vi "Lab Panel V5.12.vi"() -> ()   [LabVIEW 2013] (continued)
              n217 = local read "TEMP LA02"() -> (w247:T9)
              n218 = Bundle By Name(cluster=w247, "TL-1"=w239, "TN-1"=w238, "TL-2"=w237, "TN-2"=w236, "TL -1COUNT"=w244, "TN-1 COUNT"=w244, "TL-2 COUNT"=w244, "TN-2 COUNT"=w244) -> (w245:T9)
              n219 = Bundle(cluster=w242, "Tmp Live"=w237, "Tmp Neut"=w236) -> (w240:T2)  [unwired: 3 in]
              n220 = Bundle(cluster=w243, "Tmp Live"=w239, "Tmp Neut"=w238) -> (w241:T2)  [unwired: 3 in]
              n221 = local write "TEMP LA02"(w245) -> ()
              n222 = local write "SIG LAB02-1"(w241) -> ()
              n223 = local write "SIG LAB02-2"(w240) -> ()
            }
            frame #4 {
              w256 = 0
              n224 = local read "LAB03 TEMP"() -> (w258:T12)
              n225 = Unbundle By Name(w258) -> ("T1 Live"=w251:dbl, "T1 Neut"=w250:dbl, "T2 Live"=w249:dbl, "T2 Neut"=w248:dbl)  [unwired: 2 out]
              n226 = local read "SIG LAB03-1"() -> (w255:T2)
              n227 = local read "SIG LAB03-2"() -> (w254:T2)
              n228 = local read "TEMP LA03"() -> (w259:T9)
              n229 = Bundle By Name(cluster=w259, "TL-1"=w251, "TN-1"=w250, "TL-2"=w249, "TN-2"=w248, "TL -1COUNT"=w256, "TN-1 COUNT"=w256, "TL-2 COUNT"=w256, "TN-2 COUNT"=w256) -> (w257:T9)
              n230 = Bundle(cluster=w254, "Tmp Live"=w249, "Tmp Neut"=w248) -> (w252:T2)  [unwired: 3 in]
              n231 = Bundle(cluster=w255, "Tmp Live"=w251, "Tmp Neut"=w250) -> (w253:T2)  [unwired: 3 in]
              n232 = local write "TEMP LA03"(w257) -> ()
              n233 = local write "SIG LAB03-2"(w252) -> ()
              n234 = local write "SIG LAB03-1"(w253) -> ()
            }
            frame #5 {
              w268 = 0
              n235 = local read "LAB04 TEMP"() -> (w270:T12)
              n236 = Unbundle By Name(w270) -> ("T1 Live"=w263:dbl, "T1 Neut"=w262:dbl, "T2 Live"=w261:dbl, "T2 Neut"=w260:dbl)  [unwired: 2 out]
              n237 = local read "SIG LAB04-2"() -> (w266:T2)
              n238 = local read "SIG LAB04-1"() -> (w267:T2)
              n239 = local read "TEMP LA04"() -> (w271:T9)
              n240 = Bundle By Name(cluster=w271, "TL-1"=w263, "TN-1"=w262, "TL-2"=w261, "TN-2"=w260, "TL -1COUNT"=w268, "TN-1 COUNT"=w268, "TL-2 COUNT"=w268, "TN-2 COUNT"=w268) -> (w269:T9)
              n241 = Bundle(cluster=w266, "Tmp Live"=w261, "Tmp Neut"=w260) -> (w264:T2)  [unwired: 3 in]
              n242 = Bundle(cluster=w267, "Tmp Live"=w263, "Tmp Neut"=w262) -> (w265:T2)  [unwired: 3 in]
              n243 = local write "SIG LAB04-2"(w264) -> ()
              n244 = local write "TEMP LA04"(w269) -> ()
              n245 = local write "SIG LAB04-1"(w265) -> ()
            }
            frame #6 {
              w280 = 0
              n246 = local read "LAB05 TEMP"() -> (w282:T12)
              n247 = Unbundle By Name(w282) -> ("T1 Live"=w275:dbl, "T1 Neut"=w274:dbl, "T2 Live"=w273:dbl, "T2 Neut"=w272:dbl)  [unwired: 2 out]
              n248 = local read "SIG LAB05-2"() -> (w278:T2)
              n249 = local read "SIG LAB05-1"() -> (w279:T2)
              n250 = local read "TEMP LA05"() -> (w283:T9)
              n251 = Bundle By Name(cluster=w283, "TL-1"=w275, "TN-1"=w274, "TL-2"=w273, "TN-2"=w272, "TL -1COUNT"=w280, "TN-1 COUNT"=w280, "TL-2 COUNT"=w280, "TN-2 COUNT"=w280) -> (w281:T9)
              n252 = Bundle(cluster=w278, "Tmp Live"=w273, "Tmp Neut"=w272) -> (w276:T2)  [unwired: 3 in]
              n253 = Bundle(cluster=w279, "Tmp Live"=w275, "Tmp Neut"=w274) -> (w277:T2)  [unwired: 3 in]
              n254 = local write "SIG LAB05-2"(w276) -> ()
              n255 = local write "SIG LAB05-1"(w277) -> ()
              n256 = local write "TEMP LA05"(w281) -> ()
            }
          }
        }
        frame #8 {
          # "enable front panel, all settings done"
          n257 = property on="Tab Control 2" class="TabCtl (strict)"("DisabledEnum"=T16."Enabled" ("Disabled")) -> ()  [unwired: 2 in, 2 out]
          n258 = property on="Tab Control 2" class="TabCtl (strict)"("Value"=0) -> ()  [unwired: 2 in, 2 out]
        }
        frame #9 {
          n259 = property on="Tab Control 2" class="TabCtl (strict)"("Value"=0) -> ()  [unwired: 2 in, 2 out]
        }
      }
    }
    frame #2 {
      n260 = node-c288("loop  delay(mS)") -> (w289:T17)  [unwired: 3 in]
      n261 = timed-loop {
        timing: w289 -> [_]
        timing-out: [_] -> w288
        i -> [w315]
        stop <- w290 stop-if-true
        n262 = node-c288() -> ()  [unwired: 1 in, 1 out]
        n263 = local read "Resets Done"() -> (w294:dbl)
        n264 = Greater?(x=w294, y=1000) -> (0:w292:bool)
        n265 = local read "SELECT LAB05-2"() -> (w295:T3)
        n266 = local read "SELECT LAB05-1"() -> (w296:T3)
        n267 = local read "SELECT LAB04-2"() -> (w297:T3)
        n268 = local read "SELECT LAB03-1"() -> (w300:T3)
        n269 = local read "SELECT LAB02-2"() -> (w301:T3)
        n270 = local read "SELECT LAB01-1"() -> (w304:T3)
        n271 = local read "SELECT LAB03-2"() -> (w299:T3)
        n272 = local read "SELECT LAB01-2"() -> (w303:T3)
        n273 = local read "SELECT LAB04-1"() -> (w298:T3)
        n274 = Or(x=w292, y="stop") -> (x .or. y?=w290:bool)
        n275 = local read "SELECT LAB02-1"() -> (w302:T3)
        n276 = local read "run lab03-2"() -> (w309:bool)
        n277 = local read "run lab04-1"() -> (w308:bool)
        n278 = local read "run lab05-1"() -> (w306:bool)
        n279 = local read "run lab04-2"() -> (w307:bool)
        n280 = local read "run lab05-2"() -> (w305:bool)
        n281 = local read "run lab03-1"() -> (w310:bool)
        n282 = local read "run lab02-2"() -> (w311:bool)
        n283 = local read "run lab02-1"() -> (w312:bool)
        n284 = local read "run lab01-1"() -> (w314:bool)
        n285 = local read "run lab01-2"() -> (w313:bool)
        n286 = global write "Global display 1.vi" "stop disp"(w290) -> ()
        n287 = stacked-sequence {
          seq-local: [_ w381 _ _ _ _ _ _ _ _ _ _ _ _ _ _ _ _ _ _ _ _ _] -> [_ _ _ _ _ w2482 _ _ _ _ _ _ _ _ _ _ _ _ _ _ _ _ _]
          seq-local: [_ w380 _ _ _ _ _ _ _ _ _ _ _ _ _ _ _ _ _ _ _ _ _] -> [_ _ _ _ _ w2481 _ _ _ _ _ _ _ _ _ _ _ _ _ _ _ _ _]
          seq-local: [_ w367 _ _ _ _ _ _ _ _ _ _ _ _ _ _ _ _ _ _ _ _ _] -> [_ _ _ _ _ w2480 _ _ _ _ _ _ _ _ _ _ _ _ _ _ _ _ _]
          seq-local: [_ w366 _ _ _ _ _ _ _ _ _ _ _ _ _ _ _ _ _ _ _ _ _] -> [_ _ _ _ _ w2479 _ _ _ _ _ _ _ _ _ _ _ _ _ _ _ _ _]
          seq-local: [_ w365 _ _ _ _ _ _ _ _ _ _ _ _ _ _ _ _ _ _ _ _ _] -> [_ _ _ _ _ w2478 _ _ _ _ _ _ _ _ _ _ _ _ _ _ _ _ _]
          seq-local: [_ w364 _ _ _ _ _ _ _ _ _ _ _ _ _ _ _ _ _ _ _ _ _] -> [_ _ _ _ _ w2477 _ _ _ _ _ _ _ _ _ _ _ _ _ _ _ _ _]
          seq-local: [_ w363 _ _ _ _ _ _ _ _ _ _ _ _ _ _ _ _ _ _ _ _ _] -> [_ _ _ _ _ w2476 _ _ _ _ _ _ _ _ _ _ _ _ _ _ _ _ _]
          seq-local: [_ w362 _ _ _ _ _ _ _ _ _ _ _ _ _ _ _ _ _ _ _ _ _] -> [_ _ _ _ _ w2475 _ _ _ _ _ _ _ _ _ _ _ _ _ _ _ _ _]
          seq-local: [_ w361 _ _ _ _ _ _ _ _ _ _ _ _ _ _ _ _ _ _ _ _ _] -> [_ _ _ _ _ w2474 _ _ _ _ _ _ _ _ _ _ _ _ _ _ _ _ _]
          seq-local: [_ w360 _ _ _ _ _ _ _ _ _ _ _ _ _ _ _ _ _ _ _ _ _] -> [_ _ _ _ _ w2473 _ _ _ _ _ _ _ _ _ _ _ _ _ _ _ _ _]
          tunnel: w314 -> [_ _ w397 w645 w2072 w2502 w2817 w3304 _ _ _ _ w3847 _ w4804 _ _ w5091 w5394 w5576 _ _ _]
          tunnel: w313 -> [_ _ w396 w643 w2071 w2501 w2818 w3303 _ _ _ _ w3846 _ w4802 _ _ w5090 w5393 w5574 _ _ _]
          tunnel: w312 -> [_ _ w395 w641 w2070 w2500 w2816 w3302 _ _ _ _ w3845 _ w4800 _ _ w5089 w5392 w5573 _ _ _]
          tunnel: w311 -> [_ _ w394 w639 w2069 w2499 w2815 w3301 _ _ _ _ w3844 _ w4798 _ _ w5088 w5391 w5572 _ _ _]
          tunnel: w310 -> [_ _ w393 w637 w2068 w2498 w2814 w3300 _ _ _ _ w3843 _ w4796 _ _ w5087 w5390 w5571 _ _ _]
          tunnel: w309 -> [_ _ w392 w635 w2067 w2497 w2813 w3299 _ _ _ _ w3842 _ w4794 _ _ w5086 w5389 w5570 _ _ _]
          tunnel: w308 -> [_ _ w391 w633 w2066 w2496 w2812 w3298 _ _ _ _ w3841 _ w4792 _ _ w5085 w5388 w5569 _ _ _]
          tunnel: w307 -> [_ _ w390 w631 w2065 w2495 w2811 w3297 _ _ _ _ w3840 _ w4790 _ _ w5084 w5387 w5568 _ _ _]
          tunnel: w306 -> [_ _ w389 w629 w2064 w2494 w2810 w3296 _ _ _ _ w3839 _ w4788 _ _ w5083 w5386 w5567 _ _ _]
          tunnel: w305 -> [_ _ w388 w627 w2063 w2493 w2809 w3295 _ _ _ _ w3838 _ w4786 _ _ w5082 w5385 w5566 _ _ _]
          tunnel: w304 -> [_ _ _ w644 w2062 w2492 _ _ _ _ _ _ _ _ w4806 _ _ _ _ _ w5921 _ _]
          tunnel: w303 -> [_ _ _ w642 w2061 w2491 _ _ _ _ _ _ _ _ w4801 _ _ _ _ _ w5920 _ _]
          tunnel: w302 -> [_ _ _ w640 w2060 w2490 _ _ _ _ _ _ _ _ w4799 _ _ _ _ _ w5919 _ _]
          tunnel: w301 -> [_ _ _ w638 w2059 w2489 _ _ _ _ _ _ _ _ w4797 _ _ _ _ _ w5918 _ _]
          tunnel: w300 -> [_ _ _ w636 w2058 w2488 _ _ _ _ _ _ _ _ w4795 _ _ _ _ _ w5917 _ _]
          tunnel: w299 -> [_ _ _ w634 w2057 w2487 _ _ _ _ _ _ _ _ w4793 _ _ _ _ _ w5916 _ _]
          tunnel: w298 -> [_ _ _ w632 w2056 w2486 _ _ _ _ _ _ _ _ w4791 _ _ _ _ _ w5915 _ _]
          tunnel: w297 -> [_ _ _ w630 w2055 w2485 _ _ _ _ _ _ _ _ w4789 _ _ _ _ _ w5914 _ _]
          tunnel: w296 -> [_ _ _ w628 w2054 w2484 _ _ _ _ _ _ _ _ w4787 _ _ _ _ _ w5913 _ _]
          tunnel: w295 -> [_ _ _ w626 w2053 w2483 _ _ _ _ _ _ _ _ w4785 _ _ _ _ _ w5912 _ _]
          frame #0 {
            w323 = FALSE
            w328 = 0.5
            # "set up cycle control"
            n288 = local read "jig cycle"() -> (w327:dbl)
            n289 = local read "Amps Fail level"() -> (w321:dbl)
            n290 = local read "Simulate"() -> (w318:bool)
            n291 = Divide(x="JIG ON TIME (S)", y=w328) -> (x/y=→"on loops":dbl)
            n292 = Divide(x="JIG OFF TIME (S)", y=w328) -> (x/y=→"off loops":dbl)
            n293 = local write "Simulate IND"(w318) -> ()
            n294 = global write "Global display 3.vi" "Amps Fail"(w321) -> ()
            n295 = Increment(x=w327) -> (x+1=w326:dbl)
            n296 = local write "TEMP"(w323) -> ()
            n297 = local write "AI"(w323) -> ()
            n298 = local read "Network Directory"() -> (w320:path)
            n299 = local write "jig cycle"(w326) -> ()
            n300 = call "sub vi - check network dir v2.vi"("PATH"=w320) -> ("error"=w319:bool)  [unwired: 10 in]
            n301 = local write "network error"(w319) -> ()
            n302 = global write "Global display 3.vi" "network drive"(w319) -> ()
            n303 = event shown="[1] \"ADMIN\": Value Change" {
              selector: _ -> [_ _]
              dyn-events: _ -> [_ _]
              timeout: 10 -> [_ _]
              event Timeout {
                n304 = event-data() -> ()  [unwired: 1 in, 3 out]
              }
              event "ADMIN": Value Change {
                n305 = event-data() -> ()  [unwired: 1 in, 6 out]
                n306 = stacked-sequence {
                  seq-local: [_ w332 _] -> [_ _ w333]
                  frame #0 {
                    n307 = global write "Global 1.vi" "password"("9949") -> ()
                  }
                  frame #1 {
                    n308 = call "sub vi - password 1.vi"() -> ("RESULT"=w332:bool)  [unwired: 11 in]
                  }
                  frame #2 {
                    w335 = FALSE
                    n309 = property on="Tab Control 2" class="TabCtl (strict)"() -> ("Pages"=w339:refnum<vi>[])  [unwired: 2 in, 2 out]
                    n310 = Select(t=TRUE, s=w333, f=w335) -> (s? t:f=w334:bool)
                    n311 = Index Array(array=w339, index=8) -> (element=w337:refnum<vi>)
                    n312 = property class="Page"(reference=w337, "PageVis"=w334) -> ()  [unwired: 1 in, 2 out]
                    n313 = local write "ADMIN"(w335) -> ()
                  }
                }
              }
            }
          }
          frame #1 {
            w377 = 60.0
            # "convert temperature rise minutes to cycles"
            n314 = local read "SET LAB05-2"() -> (w341:T5)
            n315 = local read "SET LAB05-1"() -> (w343:T5)
            n316 = local read "SET LAB04-2"() -> (w345:T5)
            n317 = local read "SET LAB01-1"() -> (w359:T5)
            n318 = local read "SET LAB01-2"() -> (w357:T5)
            n319 = local read "SET LAB02-2"() -> (w353:T5)
            n320 = local read "SET LAB04-1"() -> (w347:T5)
            n321 = local read "SET LAB03-1"() -> (w351:T5)
            n322 = local read "SET LAB03-2"() -> (w349:T5)
            n323 = local read "SET LAB02-1"() -> (w355:T5)
            n324 = local read "JIG OFF TIME (S)"() -> (w382:dbl)
            n325 = local read "JIG ON TIME (S)"() -> (w383:dbl)
            n326 = Unbundle(w341) -> ("T-RISE mins"=w340:dbl)  [unwired: 4 out]
            n327 = Unbundle(w343) -> ("T-RISE mins"=w342:dbl)  [unwired: 4 out]
            n328 = Unbundle(w359) -> ("T-RISE mins"=w358:dbl)  [unwired: 4 out]
            n329 = Unbundle(w345) -> ("T-RISE mins"=w344:dbl)  [unwired: 4 out]
            n330 = Unbundle(w357) -> ("T-RISE mins"=w356:dbl)  [unwired: 4 out]
            n331 = Unbundle(w355) -> ("T-RISE mins"=w354:dbl)  [unwired: 4 out]
            n332 = Unbundle(w347) -> ("T-RISE mins"=w346:dbl)  [unwired: 4 out]
            n333 = Unbundle(w353) -> ("T-RISE mins"=w352:dbl)  [unwired: 4 out]
            n334 = Unbundle(w349) -> ("T-RISE mins"=w348:dbl)  [unwired: 4 out]
            n335 = Unbundle(w351) -> ("T-RISE mins"=w350:dbl)  [unwired: 4 out]
            n336 = Add(x=w383, y=w382) -> (x+y=w376:dbl)
            n337 = Multiply(x=w377, y=w348) -> (x*y=w372:dbl)
            n338 = Multiply(x=w377, y=w346) -> (x*y=w371:dbl)
            n339 = Multiply(x=w377, y=w344) -> (x*y=w370:dbl)
            n340 = Multiply(x=w377, y=w342) -> (x*y=w369:dbl)
            n341 = Multiply(x=w377, y=w340) -> (x*y=w368:dbl)
            n342 = Multiply(x=w377, y=w356) -> (x*y=w378:dbl)
            n343 = Multiply(x=w377, y=w350) -> (x*y=w373:dbl)
            n344 = Multiply(x=w377, y=w358) -> (x*y=w379:dbl)
            n345 = Multiply(x=w377, y=w354) -> (x*y=w375:dbl)
            n346 = Multiply(x=w377, y=w352) -> (x*y=w374:dbl)
            n347 = Divide(x=w369, y=w376) -> (x/y=w361:dbl)
            n348 = Divide(x=w370, y=w376) -> (x/y=w362:dbl)
            n349 = Divide(x=w371, y=w376) -> (x/y=w363:dbl)
            n350 = Divide(x=w368, y=w376) -> (x/y=w360:dbl)
            n351 = Divide(x=w373, y=w376) -> (x/y=w365:dbl)
            n352 = Divide(x=w379, y=w376) -> (x/y=w381:dbl)
            n353 = Divide(x=w378, y=w376) -> (x/y=w380:dbl)
            n354 = Divide(x=w375, y=w376) -> (x/y=w367:dbl)
            n355 = Divide(x=w374, y=w376) -> (x/y=w366:dbl)
            n356 = Divide(x=w372, y=w376) -> (x/y=w364:dbl)
          }
          frame #2 {
            # "control cycle loops"
            n357 = local read "JIG OFF TIME (S)"() -> (w386:dbl)
            n358 = local read "JIG ON TIME (S)"() -> (w385:dbl)
            n359 = local read "jig cycle"() -> (w399:dbl)
            n360 = local read "on loops"() -> (w401:dbl)
            n361 = local read "off loops"() -> (w400:dbl)
            n362 = Add(x=w386, y=w385) -> (x+y=w384:dbl)
            n363 = Add(x=w401, y=w400) -> (x+y=w387:dbl)
            n364 = Greater Or Equal?(x=w399, y=w387) -> (x >= y?=w398:bool)
            n365 = case shown="True" w398 {
              tunnel: w397 -> [_ w435]
              tunnel: w396 -> [_ w434]
              tunnel: w395 -> [_ w433]
              tunnel: w394 -> [_ w432]
              tunnel: w393 -> [_ w431]
              tunnel: w392 -> [_ w430]
              tunnel: w391 -> [_ w429]
              tunnel: w390 -> [_ w428]
              tunnel: w389 -> [_ w427]
              tunnel: w388 -> [_ w426]
              tunnel: w384 -> [_ w425]
              frame False {
              }
              frame True {
                # "increment cycle value and convert cycles to minutes for temp rise"
                n366 = stacked-sequence {
                  frame #0 {
                    n367 = local read "Panel #"() -> (w438:dbl)
                    n368 = Increment(x=w438) -> (x+1=w437:dbl)
                    n369 = local write "Panel #"(w437) -> ()
                  }
                  frame #1 {
                    n370 = local read "Panel #"() -> (w439:dbl)
                    n371 = Greater?(x=w439, y=5) -> (0:w441:bool)
                    n372 = case shown="True" w441 {
                      frame False {
                      }
                      frame True {
                        n373 = local write "Panel #"(1) -> ()
                      }
                    }
                  }
                }
                n374 = local read "JIG RELAY CYCLES"() -> (w424:T8)
                n375 = local read "Panel #"() -> (→"Tp Ut":dbl)
                n376 = Unbundle By Name(w424) -> ("LAB01-1"=w422:dbl, "LAB01-2"=w420:dbl, "LAB02-1"=w418:dbl, "LAB02-2"=w416:dbl, "LAB03-1"=w414:dbl, "LAB03-2"=w412:dbl, "LAB04-1"=w410:dbl, "LAB04-2"=w408:dbl, "LAB05-1"=w406:dbl, "LAB05-2"=w404:dbl)
                n377 = stacked-sequence {
                  tunnel: w435 -> [w453 _ _ _ _ _ _ _ _ _]
                  tunnel: w434 -> [_ w470 _ _ _ _ _ _ _ _]
                  tunnel: w433 -> [_ _ w487 _ _ _ _ _ _ _]
                  tunnel: w432 -> [_ _ _ w504 _ _ _ _ _ _]
                  tunnel: w431 -> [_ _ _ _ w521 _ _ _ _ _]
                  tunnel: w430 -> [_ _ _ _ _ w538 _ _ _ _]
                  tunnel: w429 -> [_ _ _ _ _ _ w555 _ _ _]
                  tunnel: w428 -> [_ _ _ _ _ _ _ w572 _ _]
                  tunnel: w427 -> [_ _ _ _ _ _ _ _ w589 _]
                  tunnel: w426 -> [_ _ _ _ _ _ _ _ _ w606]
                  tunnel: w425 -> [w450 w467 w484 w501 w518 w535 w552 w569 w586 w603]
                  tunnel: w422 -> [w444 _ _ _ _ _ _ _ _ _]
                  tunnel: [w443 _ _ _ _ _ _ _ _ _] -> w421
                  tunnel: w420 -> [_ w461 _ _ _ _ _ _ _ _]
                  tunnel: [_ w460 _ _ _ _ _ _ _ _] -> w419
                  tunnel: w418 -> [_ _ w478 _ _ _ _ _ _ _]
                  tunnel: [_ _ w477 _ _ _ _ _ _ _] -> w417
                  tunnel: w416 -> [_ _ _ w495 _ _ _ _ _ _]
                  tunnel: [_ _ _ w494 _ _ _ _ _ _] -> w415
                  tunnel: w414 -> [_ _ _ _ w512 _ _ _ _ _]
                  tunnel: [_ _ _ _ w511 _ _ _ _ _] -> w413
                  tunnel: w412 -> [_ _ _ _ _ w529 _ _ _ _]
                  tunnel: [_ _ _ _ _ w528 _ _ _ _] -> w411
                  tunnel: w410 -> [_ _ _ _ _ _ w546 _ _ _]
                  tunnel: [_ _ _ _ _ _ w545 _ _ _] -> w409
                  tunnel: w408 -> [_ _ _ _ _ _ _ w563 _ _]
                  tunnel: [_ _ _ _ _ _ _ w562 _ _] -> w407
                  tunnel: w406 -> [_ _ _ _ _ _ _ _ w580 _]
                  tunnel: [_ _ _ _ _ _ _ _ w579 _] -> w405
                  tunnel: w404 -> [_ _ _ _ _ _ _ _ _ w597]
                  tunnel: [_ _ _ _ _ _ _ _ _ w596] -> w403
                  frame #0 {
                    n378 = local read "DISP LAB01-1"() -> (w448:T4)
                    n379 = Unbundle(w448) -> ("CYCLE"=w449:dbl)  [unwired: 2 out]
                    n380 = case shown="True" w453 {
                      tunnel: w449 -> [w455 w459]
                      tunnel: [w455 w458] -> w447
                      tunnel: w444 -> [w454 w457]
                      tunnel: [w454 w456] -> w443
                      frame False {
                      }
                      frame True {
                        n381 = Increment(x=w457) -> (x+1=w456:dbl)
                        n382 = Increment(x=w459) -> (x+1=w458:dbl)
                      }
                    }
                    n383 = Multiply(x=w447, y=w450) -> (x*y=w451:dbl)
                    n384 = Divide(x=w451, y=60.0) -> (x/y=w446:dbl)
                    n385 = Bundle(cluster=w448, "CYCLE"=w447, "MINS"=w446) -> (w445:T4)  [unwired: 1 in]
                    n386 = local write "DISP LAB01-1"(w445) -> ()
                  }
                  frame #1 {
                    n387 = local read "DISP LAB01-2"() -> (w465:T4)
                    n388 = Unbundle(w465) -> ("CYCLE"=w466:dbl)  [unwired: 2 out]
                    n389 = case shown="True" w470 {
                      tunnel: w466 -> [w472 w476]
                      tunnel: [w472 w475] -> w463
                      tunnel: w461 -> [w471 w474]
                      tunnel: [w471 w473] -> w460
                      frame False {
                      }
                      frame True {
                        n390 = Increment(x=w474) -> (x+1=w473:dbl)
                        n391 = Increment(x=w476) -> (x+1=w475:dbl)
                      }
                    }
                    n392 = Multiply(x=w463, y=w467) -> (x*y=w468:dbl)
                    n393 = Divide(x=w468, y=60.0) -> (x/y=w462:dbl)
                    n394 = Bundle(cluster=w465, "CYCLE"=w463, "MINS"=w462) -> (w464:T4)  [unwired: 1 in]
                    n395 = local write "DISP LAB01-2"(w464) -> ()
                  }
                  frame #2 {
                    n396 = local read "DISP LAB02-1"() -> (w482:T4)
                    n397 = Unbundle(w482) -> ("CYCLE"=w483:dbl)  [unwired: 2 out]
                    n398 = case shown="True" w487 {
                      tunnel: [w489 w493] -> w480
                      tunnel: w483 -> [w489 w492]
                      tunnel: w478 -> [w488 w491]
                      tunnel: [w488 w490] -> w477
                      frame False {
                      }
                      frame True {
                        n399 = Increment(x=w491) -> (x+1=w490:dbl)
                        n400 = Increment(x=w492) -> (x+1=w493:dbl)
                      }
                    }
                    n401 = Multiply(x=w480, y=w484) -> (x*y=w485:dbl)
                    n402 = Divide(x=w485, y=60.0) -> (x/y=w479:dbl)
                    n403 = Bundle(cluster=w482, "CYCLE"=w480, "MINS"=w479) -> (w481:T4)  [unwired: 1 in]
                    n404 = local write "DISP LAB02-1"(w481) -> ()
                  }
                  frame #3 {
                    n405 = local read "DISP LAB02-2"() -> (w499:T4)
                    n406 = Unbundle(w499) -> ("CYCLE"=w500:dbl)  [unwired: 2 out]
                    n407 = case shown="True" w504 {
                      tunnel: [w506 w510] -> w498
                      tunnel: w500 -> [w506 w509]
                      tunnel: w495 -> [w505 w508]
                      tunnel: [w505 w507] -> w494
                      frame False {
                      }
                      frame True {
                        n408 = Increment(x=w508) -> (x+1=w507:dbl)
                        n409 = Increment(x=w509) -> (x+1=w510:dbl)
                      }
                    }
                    n410 = Multiply(x=w498, y=w501) -> (x*y=w502:dbl)
                    n411 = Divide(x=w502, y=60.0) -> (x/y=w497:dbl)
                    n412 = Bundle(cluster=w499, "CYCLE"=w498, "MINS"=w497) -> (w496:T4)  [unwired: 1 in]
                    n413 = local write "DISP LAB02-2"(w496) -> ()
                  }
                  frame #4 {
                    n414 = local read "DISP LAB03-1"() -> (w516:T4)
                    n415 = Unbundle(w516) -> ("CYCLE"=w517:dbl)  [unwired: 2 out]
                    n416 = case shown="True" w521 {
                      tunnel: [w523 w527] -> w513
                      tunnel: w517 -> [w523 w526]
                      tunnel: w512 -> [w522 w525]
                      tunnel: [w522 w524] -> w511
                      frame False {
                      }
                      frame True {
                        n417 = Increment(x=w525) -> (x+1=w524:dbl)
                        n418 = Increment(x=w526) -> (x+1=w527:dbl)
                      }
                    }
                    n419 = Multiply(x=w513, y=w518) -> (x*y=w519:dbl)
                    n420 = Divide(x=w519, y=60.0) -> (x/y=w514:dbl)
                    n421 = Bundle(cluster=w516, "CYCLE"=w513, "MINS"=w514) -> (w515:T4)  [unwired: 1 in]
                    n422 = local write "DISP LAB03-1"(w515) -> ()
                  }
                  frame #5 {
                    n423 = local read "DISP LAB03-2"() -> (w533:T4)
                    n424 = Unbundle(w533) -> ("CYCLE"=w534:dbl)  [unwired: 2 out]
                    n425 = case shown="True" w538 {
                      tunnel: [w540 w544] -> w532
                      tunnel: w534 -> [w540 w543]
                      tunnel: w529 -> [w539 w542]
                      tunnel: [w539 w541] -> w528
                      frame False {
                      }
                      frame True {
                        n426 = Increment(x=w542) -> (x+1=w541:dbl)
                        n427 = Increment(x=w543) -> (x+1=w544:dbl)
                      }
                    }
                    n428 = Multiply(x=w532, y=w535) -> (x*y=w536:dbl)
                    n429 = Divide(x=w536, y=60.0) -> (x/y=w531:dbl)
                    n430 = Bundle(cluster=w533, "CYCLE"=w532, "MINS"=w531) -> (w530:T4)  [unwired: 1 in]
                    n431 = local write "DISP LAB03-2"(w530) -> ()
                  }
                  frame #6 {
                    n432 = local read "DISP LAB04-1"() -> (w550:T4)
                    n433 = Unbundle(w550) -> ("CYCLE"=w551:dbl)  [unwired: 2 out]
                    n434 = case shown="True" w555 {
                      tunnel: [w557 w561] -> w548
                      tunnel: w551 -> [w557 w560]
                      tunnel: w546 -> [w556 w559]
                      tunnel: [w556 w558] -> w545
                      frame False {
                      }
                      frame True {
                        n435 = Increment(x=w559) -> (x+1=w558:dbl)
                        n436 = Increment(x=w560) -> (x+1=w561:dbl)
                      }
                    }
                    n437 = Multiply(x=w548, y=w552) -> (x*y=w553:dbl)
                    n438 = Divide(x=w553, y=60.0) -> (x/y=w547:dbl)
                    n439 = Bundle(cluster=w550, "CYCLE"=w548, "MINS"=w547) -> (w549:T4)  [unwired: 1 in]
                    n440 = local write "DISP LAB04-1"(w549) -> ()
                  }
                  frame #7 {
                    n441 = local read "DISP LAB04-2"() -> (w567:T4)
                    n442 = Unbundle(w567) -> ("CYCLE"=w568:dbl)  [unwired: 2 out]
                    n443 = case shown="True" w572 {
                      tunnel: [w574 w578] -> w565
                      tunnel: w568 -> [w574 w577]
                      tunnel: w563 -> [w573 w576]
                      tunnel: [w573 w575] -> w562
                      frame False {
                      }
                      frame True {
                        n444 = Increment(x=w576) -> (x+1=w575:dbl)
                        n445 = Increment(x=w577) -> (x+1=w578:dbl)
                      }
                    }
                    n446 = Multiply(x=w565, y=w569) -> (x*y=w571:dbl)
                    n447 = Divide(x=w571, y=60.0) -> (x/y=w564:dbl)
                    n448 = Bundle(cluster=w567, "CYCLE"=w565, "MINS"=w564) -> (w566:T4)  [unwired: 1 in]
                    n449 = local write "DISP LAB04-2"(w566) -> ()
                  }
                  frame #8 {
                    n450 = local read "DISP LAB05-1"() -> (w584:T4)
                    n451 = Unbundle(w584) -> ("CYCLE"=w585:dbl)  [unwired: 2 out]
                    n452 = case shown="True" w589 {
                      tunnel: [w591 w595] -> w582
                      tunnel: w585 -> [w591 w594]
                      tunnel: w580 -> [w590 w593]
                      tunnel: [w590 w592] -> w579
                      frame False {
                      }
                      frame True {
                        n453 = Increment(x=w593) -> (x+1=w592:dbl)
                        n454 = Increment(x=w594) -> (x+1=w595:dbl)
                      }
                    }
                    n455 = Multiply(x=w582, y=w586) -> (x*y=w587:dbl)
                    n456 = Divide(x=w587, y=60.0) -> (x/y=w581:dbl)
                    n457 = Bundle(cluster=w584, "CYCLE"=w582, "MINS"=w581) -> (w583:T4)  [unwired: 1 in]
                    n458 = local write "DISP LAB05-1"(w583) -> ()
                  }
                  frame #9 {
                    n459 = local read "DISP LAB05-2"() -> (w602:T4)
                    n460 = Unbundle(w602) -> ("CYCLE"=w601:dbl)  [unwired: 2 out]
                    n461 = case shown="True" w606 {
                      tunnel: [w608 w612] -> w600
                      tunnel: w601 -> [w608 w611]
                      tunnel: w597 -> [w607 w610]
                      tunnel: [w607 w609] -> w596
                      frame False {
                      }
                      frame True {
                        n462 = Increment(x=w610) -> (x+1=w609:dbl)
                        n463 = Increment(x=w611) -> (x+1=w612:dbl)
                      }
                    }
                    n464 = Multiply(x=w600, y=w603) -> (x*y=w604:dbl)
                    n465 = Divide(x=w604, y=60.0) -> (x/y=w599:dbl)
                    n466 = Bundle(cluster=w602, "CYCLE"=w600, "MINS"=w599) -> (w598:T4)  [unwired: 1 in]
                    n467 = local write "DISP LAB05-2"(w598) -> ()
                  }
                }
                n468 = local write "jig cycle"(0) -> ()
                n469 = Bundle By Name(cluster=w424, "LAB01-1"=w421, "LAB01-2"=w419, "LAB02-1"=w417, "LAB02-2"=w415, "LAB03-1"=w413, "LAB03-2"=w411, "LAB04-1"=w409, "LAB04-2"=w407, "LAB05-1"=w405, "LAB05-2"=w403) -> (w423:T8)
                n470 = local write "JIG RELAY CYCLES"(w423) -> ()
              }
            }
          }
          frame #3 {
            # "START & STOP test RUN switch change, start test if true and stop test if false"
            n471 = Get Date/Time In Seconds() -> (seconds since 1Jan1904=w624:timestamp)
            n472 = local read "C drive data root dir"() -> (w617:path)
            n473 = Format Date/Time String(time format string (%c)="%b\\%a%d", seconds (now)=w624) -> (date/time string=w648:string)  [unwired: 1 in]
            n474 = Format Date/Time String(time format string (%c)="%H%M", seconds (now)=w624) -> (date/time string=w646:string)  [unwired: 1 in]
            n475 = Format Date/Time String(time format string (%c)="LabPanel%Y", seconds (now)=w624) -> (date/time string=w623:string)  [unwired: 1 in]
            n476 = Path To String(path=w617) -> (string=w620:string)
            n477 = global write "Global 1.vi" "C drive root path"(w617) -> ()
            n478 = local read "Ref deg C"() -> (w613:dbl)
            n479 = Concatenate Strings(w620, "\\") -> (w618:string)
            n480 = event shown="[1] \"RUN LAB01-1\": Value Change" {
              selector: _ -> [_ _ _ _ _ _ _ _ _ _ _]
              dyn-events: _ -> [_ _ _ _ _ _ _ _ _ _ _]
              timeout: 10 -> [_ _ _ _ _ _ _ _ _ _ _]
              tunnel: w618 -> [_ w661 w801 w942 w1082 w1222 w1362 w1502 w1642 w1782 w1923]
              tunnel: w648 -> [_ w660 w800 w941 w1081 w1221 w1361 w1501 w1641 w1781 w1922]
              tunnel: w646 -> [_ w658 w799 w940 w1080 w1220 w1360 w1500 w1640 w1780 w1921]
              tunnel: w644 -> [_ w659 _ _ _ _ _ _ _ _ _]
              tunnel: w645 -> [_ _ _ _ _ _ _ _ _ _ _]
              tunnel: w643 -> [_ _ _ _ _ _ _ _ _ _ _]
              tunnel: w642 -> [_ _ w798 _ _ _ _ _ _ _ _]
              tunnel: w641 -> [_ _ _ _ _ _ _ _ _ _ _]
              tunnel: w640 -> [_ _ _ w939 _ _ _ _ _ _ _]
              tunnel: w639 -> [_ _ _ _ _ _ _ _ _ _ _]
              tunnel: w638 -> [_ _ _ _ w1079 _ _ _ _ _ _]
              tunnel: w637 -> [_ _ _ _ _ _ _ _ _ _ _]
              tunnel: w636 -> [_ _ _ _ _ w1219 _ _ _ _ _]
              tunnel: w635 -> [_ _ _ _ _ _ _ _ _ _ _]
              tunnel: w634 -> [_ _ _ _ _ _ w1359 _ _ _ _]
              tunnel: w633 -> [_ _ _ _ _ _ _ _ _ _ _]
              tunnel: w632 -> [_ _ _ _ _ _ _ w1499 _ _ _]
              tunnel: w631 -> [_ _ _ _ _ _ _ _ _ _ _]
              tunnel: w630 -> [_ _ _ _ _ _ _ _ w1639 _ _]
              tunnel: w629 -> [_ _ _ _ _ _ _ _ _ _ _]
              tunnel: w628 -> [_ _ _ _ _ _ _ _ _ w1779 _]
              tunnel: w627 -> [_ _ _ _ _ _ _ _ _ _ _]
              tunnel: w626 -> [_ _ _ _ _ _ _ _ _ _ w1920]
              tunnel: w623 -> [_ w657 w797 w938 w1078 w1218 w1358 w1498 w1638 w1778 w1919]
              tunnel: [_ w656 w796 w937 w1077 w1217 w1357 w1497 w1637 w1777 w1918] -> w621
              tunnel: "RESET CYCLES TO ZERO?" -> [_ w655 w794 w935 w1075 w1215 w1355 w1495 w1635 w1775 w1916]
              tunnel: "YES" -> [_ w654 w793 w934 w1074 w1214 w1354 w1494 w1634 w1774 w1915]
              tunnel: "NO" -> [_ w653 w792 w933 w1073 w1213 w1353 w1493 w1633 w1773 w1914]
              tunnel: w613 -> [_ w650 w791 w931 w1072 w1212 w1352 w1492 w1632 w1772 w1912]
              event Timeout {
                n481 = event-data() -> ()  [unwired: 1 in, 3 out]
              }
              event "RUN LAB01-1": Value Change {
                n482 = event-data() -> ("NewVal"=w651:bool)  [unwired: 1 in, 5 out]
                n483 = local read "SIG LAB01-1"() -> (w652:T2)
                n484 = local write "run lab01-1"(w651) -> ()
                n485 = case shown="True" w651 {
                  tunnel: w661 -> [_ w699]
                  tunnel: w660 -> [_ w698]
                  tunnel: w659 -> [w663 w697]
                  tunnel: w658 -> [_ w696]
                  tunnel: w657 -> [_ w695]
                  tunnel: [w662 w694] -> w656
                  tunnel: w655 -> [_ w693]
                  tunnel: w654 -> [_ w692]
                  tunnel: w653 -> [_ w691]
                  tunnel: w652 -> [_ w690]
                  tunnel: w650 -> [_ w689]
                  frame False {
                    # "stop test"
                    n486 = stacked-sequence {
                      tunnel: w663 -> [_ w675 _]
                      tunnel: [_ w667 _] -> w662
                      frame #0 {
                        n487 = local read "DISP LAB01-1"() -> (w666:T4)
                        n488 = Bundle(cluster=w666, "STATUS"="STOP") -> (w664:T4)  [unwired: 2 in]
                        n489 = local write "DISP LAB01-1"(w664) -> ()
                      }
                      frame #1 {
                        n490 = local read "DISP LAB01-1"() -> (w674:T4)
                        n491 = Unbundle(w674) -> ("CYCLE"=w672:dbl, "MINS"=w673:dbl)  [unwired: 1 out]
                        n492 = case shown="\"CYCLE TEST\"" w675 {
                          tunnel: w673 -> [_ _ w682]
                          tunnel: w672 -> [w680 w681 _]
                          tunnel: [w680 w681 w682] -> w671
                          frame "CHART TEST", Default {
                          }
                          frame "CYCLE TEST" {
                          }
                          frame "T-RISE TEST" {
                          }
                        }
                        n493 = local read "TDMS LAB01-1"() -> (w679:refnum<k34>)
                        n494 = Build Array("STOPPED") -> (w676:string[])
                        n495 = Build Array(w671) -> (w670:dbl[])
                        n496 = TDMS Write(0:w679, 5:"TEST RESULT", 7:w676, 9:w670) -> (4:w668:refnum<k34>, 15:w669:errorcluster)  [unwired: 2 in, 2 out]
                        n497 = TDMS Close(8:w669, 11:w668) -> (0:w667:errorcluster)  [unwired: 1 out]
                      }
                      frame #2 {
                        n498 = stacked-sequence {
                          tunnel: "LAB01-1" -> [w685 w687]
                          frame #0 {
                            n499 = call "sub vi - defrag tdms v1.vi"("panel id"=w685) -> ("error out"=w684:errorcluster)  [unwired: 10 in]
                            n500 = local write "data file error"(w684) -> ()
                          }
                          frame #1 {
                            n501 = call "Save data file (stop) v3.vi"("panel id"=w687) -> ("network file save error"=w686:errorcluster)  [unwired: 9 in, 1 out]
                            n502 = local write "RESULT LAB01-1"(FALSE) -> ()
                            n503 = local write "data file error"(w686) -> ()
                          }
                        }
                      }
                    }
                  }
                  frame True {
                    n504 = stacked-sequence {
                      seq-local: [w701 _] -> [_ w705]
                      tunnel: w699 -> [_ w715]
                      tunnel: w698 -> [_ w714]
                      tunnel: w697 -> [_ w713]
                      tunnel: w696 -> [_ w712]
                      tunnel: w695 -> [_ w711]
                      tunnel: [_ w710] -> w694
                      tunnel: w693 -> [_ w709]
                      tunnel: w692 -> [_ w708]
                      tunnel: w691 -> [_ w707]
                      tunnel: w690 -> [w703 w706]
                      tunnel: w689 -> [_ w704]
                      frame #0 {
                        n505 = Unbundle(w703) -> ("AMPS"=w702:dbl)  [unwired: 4 out]
                        n506 = call "Check For Amps on v1.vi"("ID"="LAB01-1", "amps"=w702) -> ("amps"=w701:bool)  [unwired: 9 in]
                      }
                      frame #1 {
                        n507 = case shown="True" w705 {
                          tunnel: w715 -> [_ w728]
                          tunnel: w714 -> [_ w727]
                          tunnel: w713 -> [_ w726]
                          tunnel: w712 -> [_ w725]
                          tunnel: w711 -> [_ w724]
                          tunnel: [errorcluster {"status"=FALSE, "code"=0, "source"=""} ("error out") w723] -> w710
                          tunnel: w709 -> [_ w722]
                          tunnel: w708 -> [_ w721]
                          tunnel: w707 -> [_ w720]
                          tunnel: w706 -> [_ w719]
                          tunnel: w704 -> [_ w718]
                          frame False {
                            w716 = FALSE
                            n508 = local write "RUN LAB01-1"(w716) -> ()
                            n509 = local write "run lab01-1"(w716) -> ()
                          }
                          frame True {
                            n510 = stacked-sequence {
                              seq-local: [w729 _ _ _ _] -> [_ w750 _ _ _]
                              tunnel: w728 -> [w734 _ _ _ _]
                              tunnel: w727 -> [w730 _ _ _ _]
                              tunnel: w726 -> [w744 _ _ _ _]
                              tunnel: w725 -> [w737 _ _ _ _]
                              tunnel: w724 -> [w732 _ _ _ _]
                              tunnel: [_ w751 _ _ _] -> w723
                              tunnel: w722 -> [_ _ _ w772 _]
                              tunnel: w721 -> [_ _ _ w782 _]
                              tunnel: w720 -> [_ _ _ w781 _]
                              tunnel: w719 -> [_ _ _ _ _]
                              tunnel: w718 -> [_ _ _ _ w788]
                              frame #0 {
                                w731 = "\\"
                                n511 = case shown="\"CHART TEST\", Default" w744 {
                                tunnel: ["L01-1-CHART TEST-" "L01-1-CYCLE TEST-" "L01-1-T-RISE TEST-"] -> w740
                                frame "CHART TEST", Default {
                                }
                                frame "CYCLE TEST" {
                                }
                                frame "T-RISE TEST" {
                                }
                                }
                                n512 = local read "SET LAB01-1"() -> (w739:T5)
                                n513 = Unbundle(w739) -> ("DESCRIPTION"=w738:string)  [unwired: 4 out]
                                n514 = Concatenate Strings(w734, "\\", w732, w731, w730, w731) -> (w741:string)
                                n515 = String To Path(string=w741) -> (path=w743:path)
                                n516 = Concatenate Strings(w741, w740, w738, "-", w737, ".tdms") -> (w729:string)
                                n517 = Create Folder(path (use dialog)=w743) -> (error out=w742:errorcluster)  [unwired: 2 in, 2 out]
                                n518 = call <vilib>:"Clear Errors.vi"("error in (no error)"=w742) -> ()  [unwired: 6 in, 1 out]
                                n519 = global write "Global 1.vi" "LAB01-1 FILE"(w729) -> ()
                              }
                              frame #1 {
                                (unwired) FALSE
                                n520 = String To Path(string=w750) -> (path=w748:path)
                                n521 = TDMS Open(6:FALSE, 10:T20."create or replace" ("operation (0:open)"), 11:w748) -> (0:w751:errorcluster, 3:→"TDMS LAB01-1":refnum<k34>)  [unwired: 4 in]
                              }
                              frame #2 {
                                n522 = local read "TDMS LAB01-1"() -> (w770:refnum<k34>)
                                n523 = local read "SET LAB01-1"() -> (w759:T5)
                                n524 = Build Array("Testers Name", "Description", "Set Test Cycles", "T-Rise minutes", "T-Rise Deg C") -> (w760:string[])
                                n525 = Unbundle(w759) -> ("NAME"=w758:string, "DESCRIPTION"=w757:string, "CYCLES"=w756:dbl, "T-RISE mins"=w755:dbl, "T-RISE deg C"=w754:dbl)
                                n526 = Number To Decimal String(number=w756) -> (decimal integer string=w769:string)  [unwired: 1 in]
                                n527 = Number To Decimal String(number=w755) -> (decimal integer string=w768:string)  [unwired: 1 in]
                                n528 = Number To Decimal String(number=w754) -> (decimal integer string=w767:string)  [unwired: 1 in]
                                n529 = Build Array(w758, w757, w769, w768, w767) -> (w766:string[])
                                n530 = TDMS Set Properties(5:w766, 7:w760, 11:w770) -> ()  [unwired: 3 in, 4 out]
                              }
                              frame #3 {
                                n531 = local read "DISP LAB01-1"() -> (w780:T4)
                                n532 = Concatenate Strings("LAB01-1  ", w772) -> (w771:string)
                                n533 = Two Button Dialog(message=w771, 1:w781, 2:w782) -> (T button?=w774:bool)
                                n534 = case shown="True" w774 {
                                tunnel: w780 -> [w785 w786]
                                tunnel: [w785 w786] -> w779
                                tunnel: [w784 w787] -> w778
                                tunnel: [w783 w787] -> w777
                                frame False {
                                n535 = Unbundle(w785) -> ("CYCLE"=w784:dbl, "MINS"=w783:dbl)  [unwired: 1 out]
                                }
                                frame True {
                                w787 = 0.0
                                }
                                }
                                n536 = Bundle(cluster=w779, "CYCLE"=w778, "MINS"=w777, "STATUS"="RUN") -> (w776:T4)
                                n537 = local write "DISP LAB01-1"(w776) -> ()
                              }
                              frame #4 {
                                n538 = local read "TEMP START LAB01-1"() -> (w790:cluster{"TL":dbl, "TN":dbl})
                                n539 = Bundle(cluster=w790, "TL"=w788, "TN"=w788) -> (w789:cluster{"TL":dbl, "TN":dbl})
                                n540 = local write "TEMP START LAB01-1"(w789) -> ()
                              }
                            }
                          }
                        }
                      }
                    }
                  }
                }
              }
              event "RUN LAB01-2": Value Change {
                n541 = event-data() -> ("NewVal"=w795:bool)  [unwired: 1 in, 5 out]
                n542 = local write "run lab01-2"(w795) -> ()
                n543 = case shown="True" w795 {
                  tunnel: w801 -> [_ w839]
                  tunnel: w800 -> [_ w838]
                  tunnel: w798 -> [w803 w837]
                  tunnel: w799 -> [_ w836]
                  tunnel: w797 -> [_ w835]
                  tunnel: [w802 w834] -> w796
                  tunnel: w794 -> [_ w833]
                  tunnel: w793 -> [_ w832]
                  tunnel: w792 -> [_ w831]
                  tunnel: w791 -> [_ w829]
                  frame False {
                    # "stop test"
                    n544 = stacked-sequence {
                      tunnel: w803 -> [w812 _]
                      tunnel: [w804 _] -> w802
                      frame #0 {
                        n545 = local read "DISP LAB01-2"() -> (w811:T4)
                        n546 = Unbundle(w811) -> ("CYCLE"=w809:dbl, "MINS"=w810:dbl)  [unwired: 1 out]
                        n547 = case shown="\"CHART TEST\", Default" w812 {
                          tunnel: w810 -> [_ _ w819]
                          tunnel: w809 -> [w817 w818 _]
                          tunnel: [w817 w818 w819] -> w808
                          frame "CHART TEST", Default {
                          }
                          frame "CYCLE TEST" {
                          }
                          frame "T-RISE TEST" {
                          }
                        }
                        n548 = local read "TDMS LAB01-2"() -> (w816:refnum<k34>)
                        n549 = Build Array("STOPPED") -> (w813:string[])
                        n550 = Build Array(w808) -> (w807:dbl[])
                        n551 = TDMS Write(0:w816, 5:"TEST RESULT", 7:w813, 9:w807) -> (4:w805:refnum<k34>, 15:w806:errorcluster)  [unwired: 2 in, 2 out]
                        n552 = TDMS Close(8:w806, 11:w805) -> (0:w804:errorcluster)  [unwired: 1 out]
                      }
                      frame #1 {
                        n553 = local read "DISP LAB01-2"() -> (w823:T4)
                        n554 = stacked-sequence {
                          tunnel: "LAB01-2" -> [w825 w827]
                          frame #0 {
                            n555 = call "sub vi - defrag tdms v1.vi"("panel id"=w825) -> ("error out"=w824:errorcluster)  [unwired: 10 in]
                            n556 = local write "data file error"(w824) -> ()
                          }
                          frame #1 {
                            n557 = call "Save data file (stop) v3.vi"("panel id"=w827) -> ("network file save error"=w826:errorcluster)  [unwired: 9 in, 1 out]
                            n558 = local write "RESULT LAB01-2"(FALSE) -> ()
                            n559 = local write "data file error"(w826) -> ()
                          }
                        }
                        n560 = Bundle(cluster=w823, "STATUS"="STOP") -> (w821:T4)  [unwired: 2 in]
                        n561 = local write "DISP LAB01-2"(w821) -> ()
                      }
                    }
                  }
                  frame True {
                    n562 = local read "SIG LAB01-2"() -> (w830:T2)
                    n563 = stacked-sequence {
                      seq-local: [w841 _] -> [_ w845]
                      tunnel: w839 -> [_ w855]
                      tunnel: w838 -> [_ w854]
                      tunnel: w837 -> [_ w853]
                      tunnel: w836 -> [_ w852]
                      tunnel: w835 -> [_ w851]
                      tunnel: [_ w850] -> w834
                      tunnel: w833 -> [_ w849]
                      tunnel: w832 -> [_ w848]
                      tunnel: w831 -> [_ w847]
                      tunnel: w830 -> [w840 w846]
                      tunnel: w829 -> [_ w844]
                      frame #0 {
                        n564 = Unbundle(w840) -> ("AMPS"=w843:dbl)  [unwired: 4 out]
                        n565 = call "Check For Amps on v1.vi"("ID"="LAB01-2", "amps"=w843) -> ("amps"=w841:bool)  [unwired: 9 in]
                      }
                      frame #1 {
                        n566 = case shown="True" w845 {
                          tunnel: w855 -> [_ w868]
                          tunnel: w854 -> [_ w867]
                          tunnel: w853 -> [_ w866]
                          tunnel: w852 -> [_ w865]
                          tunnel: w851 -> [_ w864]
                          tunnel: [errorcluster {"status"=FALSE, "code"=0, "source"=""} ("error out") w863] -> w850
                          tunnel: w849 -> [_ w862]
                          tunnel: w848 -> [_ w861]
                          tunnel: w847 -> [_ w860]
                          tunnel: w846 -> [_ w859]
                          tunnel: w844 -> [_ w858]
                          frame False {
                            w856 = FALSE
                            n567 = local write "RUN LAB01-2"(w856) -> ()
                            n568 = local write "run lab01-2"(w856) -> ()
                          }
                          frame True {
                            n569 = stacked-sequence {
                              seq-local: [w869 _ _ _ _] -> [_ w893 _ _ _]
                              tunnel: w868 -> [w874 _ _ _ _]
                              tunnel: w867 -> [w871 _ _ _ _]
                              tunnel: w866 -> [w884 _ _ _ _]
                              tunnel: w865 -> [w877 _ _ _ _]
                              tunnel: w864 -> [w872 _ _ _ _]
                              tunnel: [_ w888 _ _ _] -> w863
                              tunnel: w862 -> [_ _ _ w915 _]
                              tunnel: w861 -> [_ _ _ w914 _]
                              tunnel: w860 -> [_ _ _ w913 _]
                              tunnel: w859 -> [_ _ _ _ _]
                              tunnel: w858 -> [_ _ _ _ w928]
                              frame #0 {
                                w870 = "\\"
                                n570 = local read "SET LAB01-2"() -> (w879:T5)
                                n571 = case shown="\"CYCLE TEST\"" w884 {
                                tunnel: ["L01-2-CHART TEST-" "L01-2-CYCLE TEST-" "L01-2-T-RISE TEST-"] -> w880
                                frame "CHART TEST", Default {
                                }
                                frame "CYCLE TEST" {
                                }
                                frame "T-RISE TEST" {
                                }
                                }
                                n572 = Unbundle(w879) -> ("DESCRIPTION"=w878:string)  [unwired: 4 out]
                                n573 = Concatenate Strings(w874, "\\", w872, w870, w871, w870) -> (w881:string)
                                n574 = String To Path(string=w881) -> (path=w883:path)
                                n575 = Concatenate Strings(w881, w880, w878, "-", w877, ".tdms") -> (w869:string)
                                n576 = Create Folder(path (use dialog)=w883) -> (error out=w882:errorcluster)  [unwired: 2 in, 2 out]
                                n577 = call <vilib>:"Clear Errors.vi"("error in (no error)"=w882) -> ()  [unwired: 6 in, 1 out]
                                n578 = global write "Global 1.vi" "LAB01-2 FILE"(w869) -> ()
                              }
                              frame #1 {
                                (unwired) FALSE
